vi "测试报告摘要4.vi"(8 "打印?":bool, 10 "试验时间":timestamp) -> ()   [LabVIEW 2010]
uses:
  <vilib>/Utility/NIReport.llb/NI_report.lvclass
  全局量/试验配置信息.vi
  <vilib>/Utility/NIReport.llb/Append Report Text (str wrap).vi
  全局量/自动测试结果.vi
  <vilib>/addons/_office/word.llb/Word Easy Table (str).vi
  <vilib>/addons/_office/NI_ReportGenerationToolkit.lvlib
panel:
  in  "序号":i32
  out "XY图":cluster{"Y":dbl[], "Y":dbl[]}[](graph)
  # "T：打印\nF：保存"
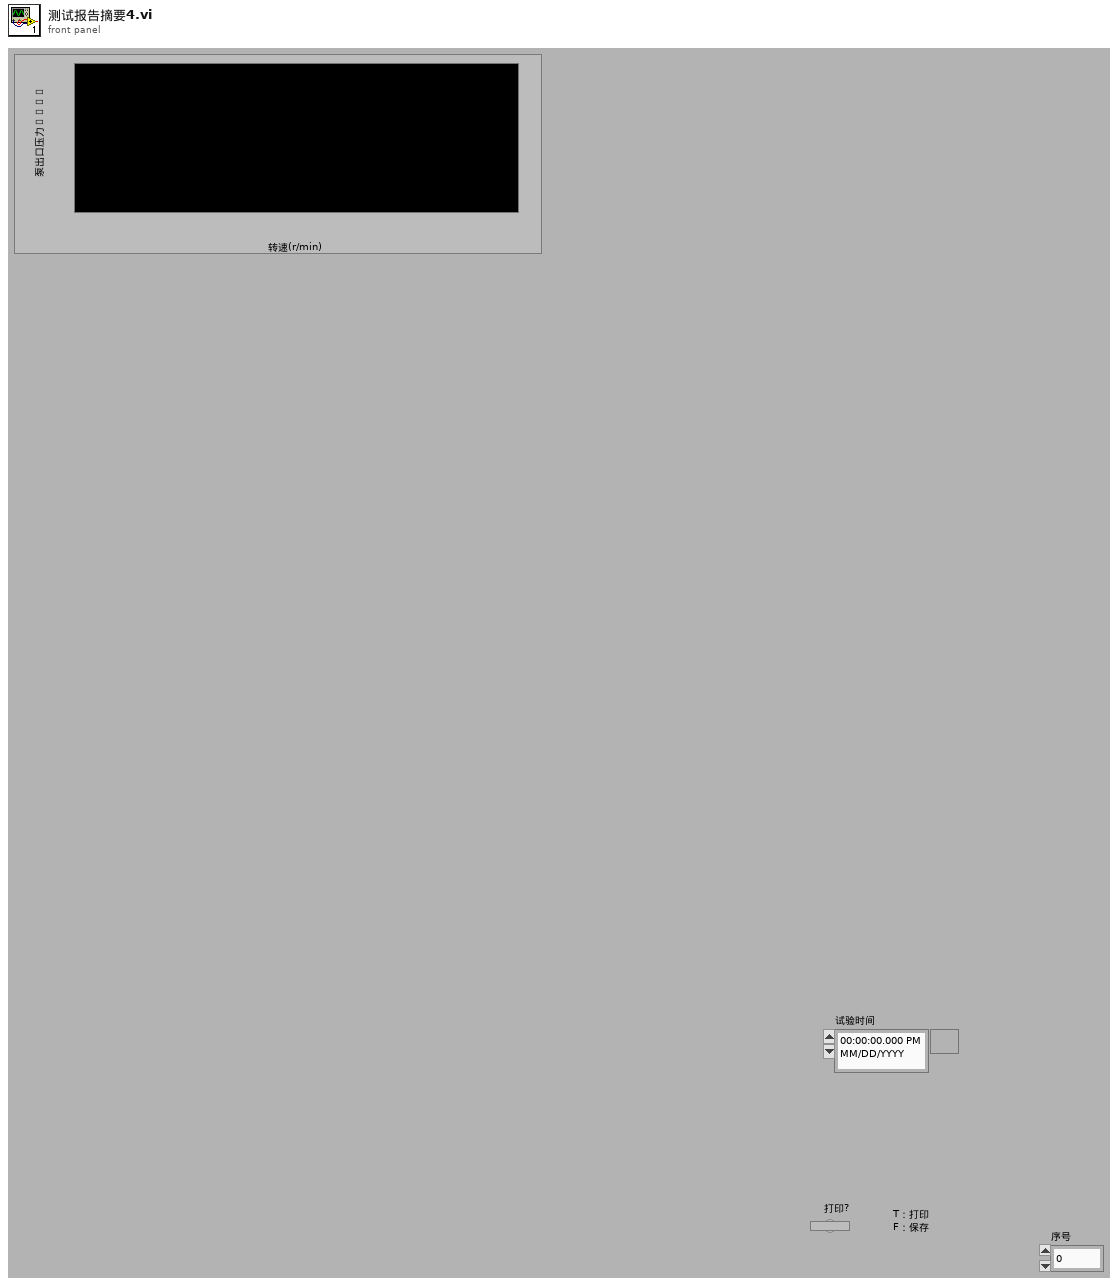
[diagram p1: front panel]
types:
  T1 = cluster{"position (Excel)":cluster{"row":i32, "column":i32}, "name (Excel)":string, "bookmark (Word)":string}
  T2 = enum16{"maximized", "minimized", "normal", "no change"}
  T3 = enum16{"Standard Report", "HTML", "Word", "Excel"}
  T4 = cluster{"报告编号":string, "控制板编号":string, "控制板类型":string, "测试人员":string, "测试地点":string, string, u64, "spreadsheet string":string, "spreadsheet string":string, "spreadsheet string":string, "spreadsheet string":string}
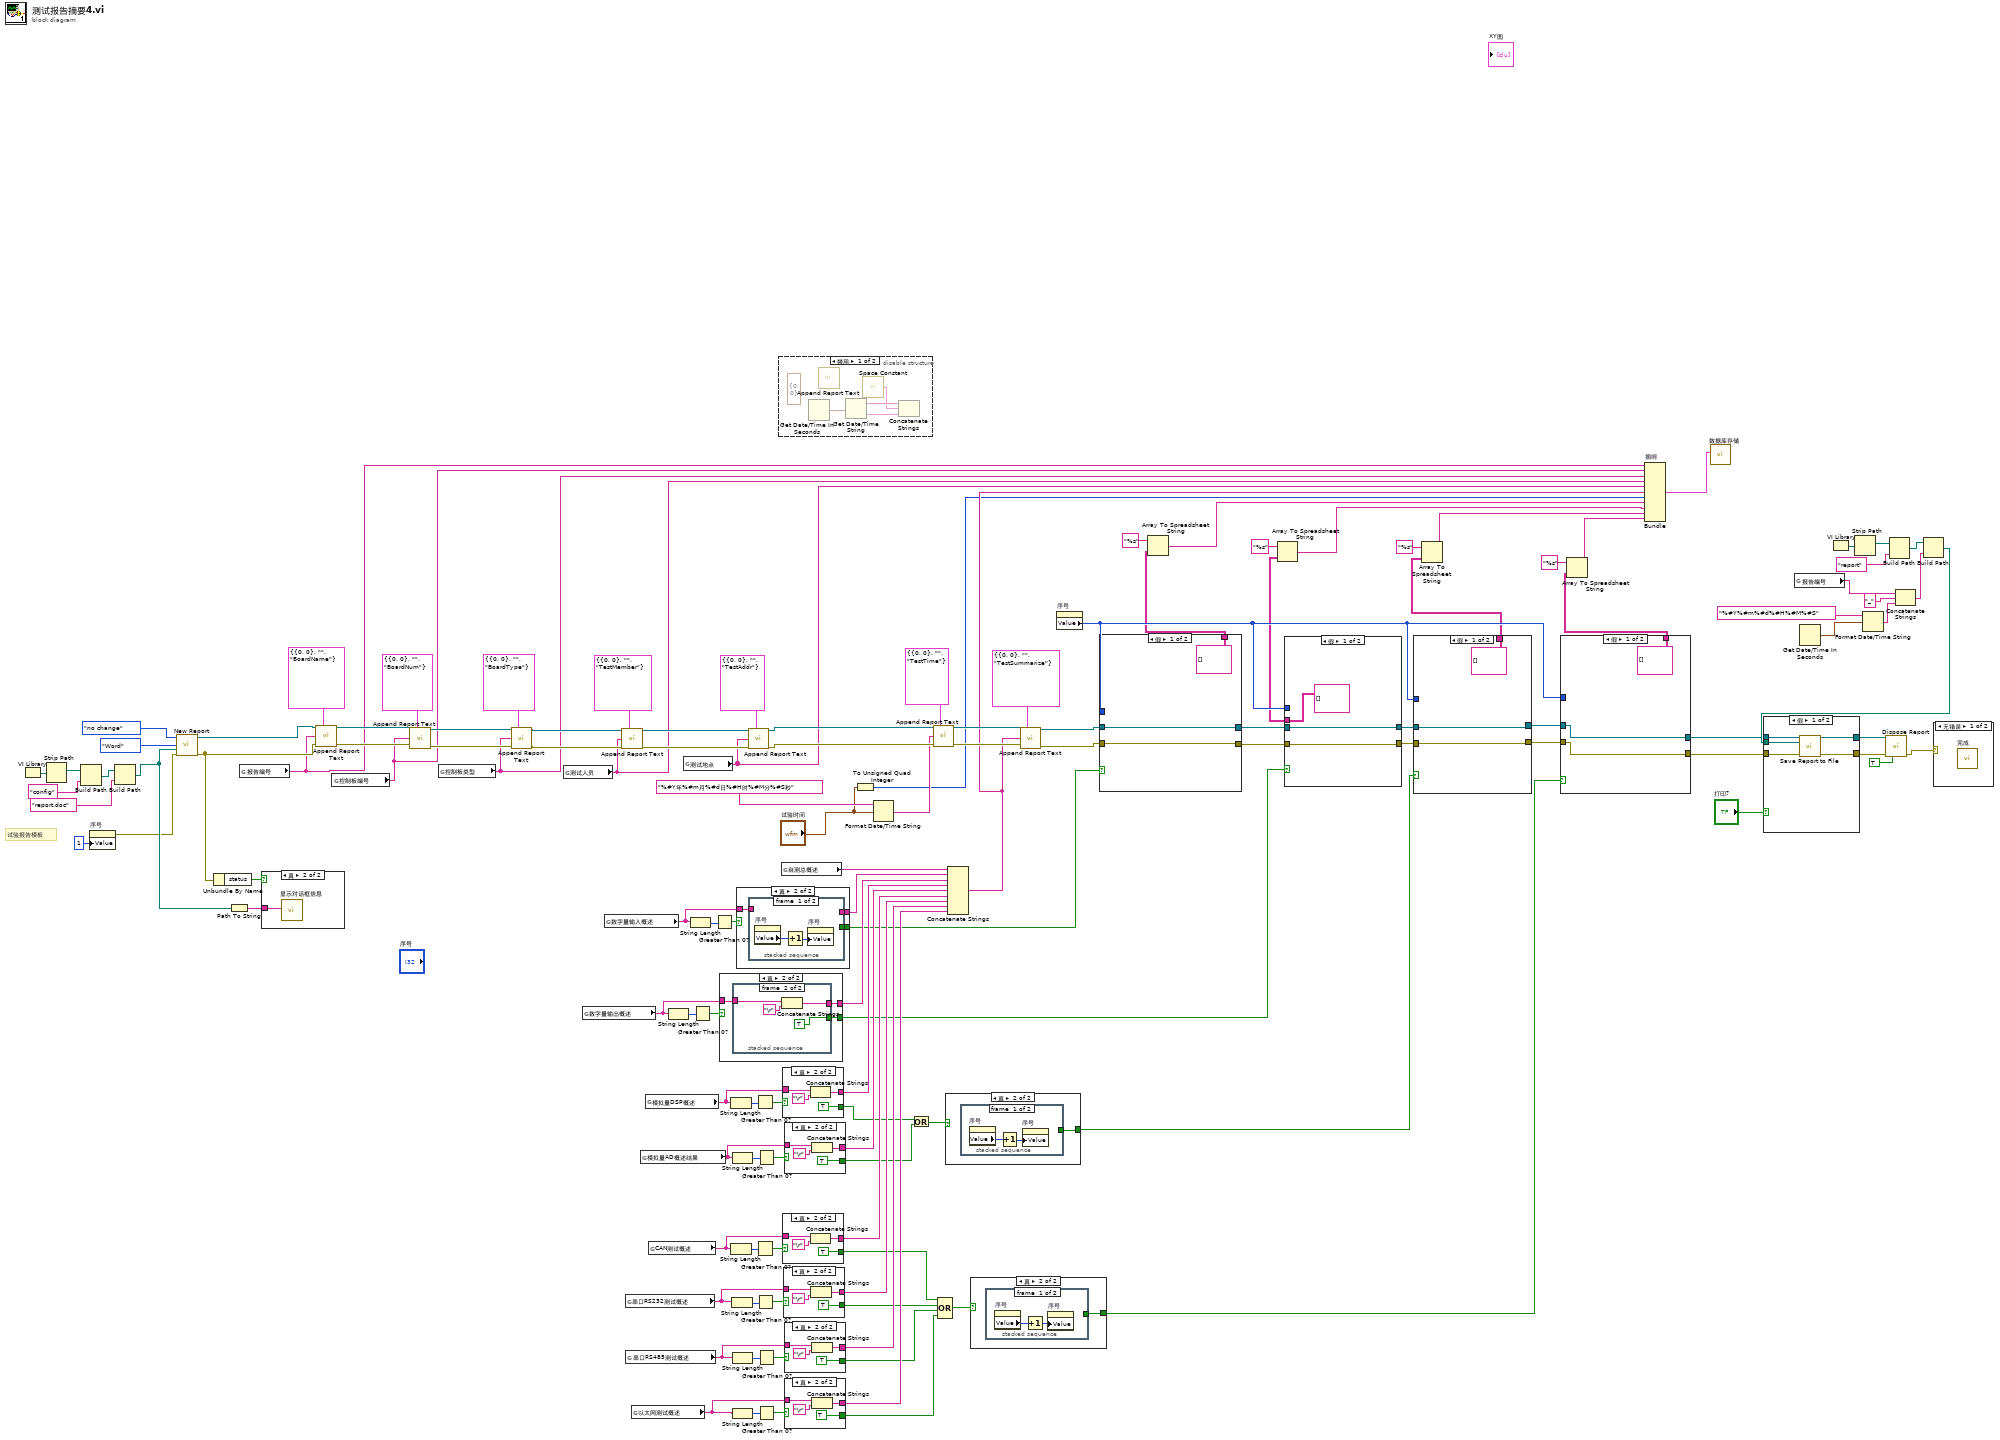
[diagram p0: block diagram]
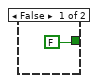
[diagram p2: hidden frame]
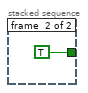
[diagram p3: hidden frame]
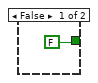
[diagram p4: hidden frame]
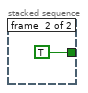
[diagram p5: hidden frame]
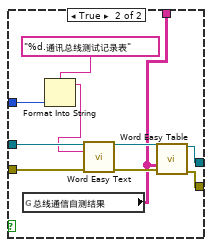
[diagram p6: hidden frame]
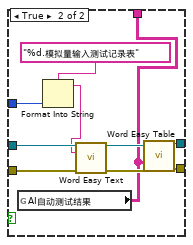
[diagram p7: hidden frame]
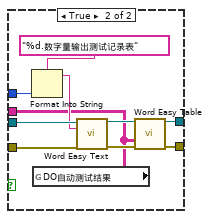
[diagram p8: hidden frame]
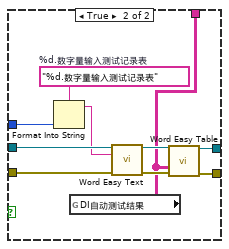
[diagram p9: hidden frame]
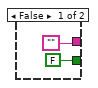
[diagram p10: hidden frame]
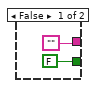
[diagram p11: hidden frame]
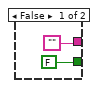
[diagram p12: hidden frame]
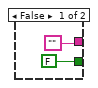
[diagram p13: hidden frame]
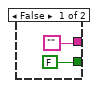
[diagram p14: hidden frame]
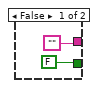
[diagram p15: hidden frame]
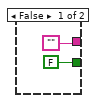
[diagram p16: hidden frame]
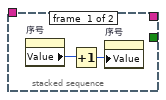
[diagram p17: hidden frame]
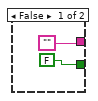
[diagram p18: hidden frame]
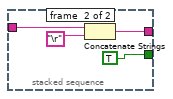
[diagram p19: hidden frame]
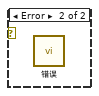
[diagram p20: hidden frame]
diagram:
  # "试验报告模板"
  n1 = VI Library() -> (path=w123:path)
  n2 = Strip Path(path=w123) -> (stripped path=w120:path)  [unwired: 1 out]
  n3 = Build Path(base path=w120, name or relative path="config") -> (appended path=w122:path)
  n4 = property on="序号" class="DigNum (严格)"("Value"=1 ("序号")) -> (error out=w40:errorcluster)  [unwired: 2 in, 1 out]
  n5 = Build Path(base path=w122, name or relative path="report.doc") -> (appended path=w126:path)
  n6 = call <vilib>:"New Report.vi"("window state (normal)"=T2."no change", "report type"=T3."Word", "template (empty)"=w126, "error in (no error)"=w40) -> ("report out"=w117:refnum<class "NI_report.lvclass">, "error out"=w116:errorcluster)  [unwired: 10 in]
  n7 = Unbundle By Name(w116) -> ("status"=w128:bool)
  n8 = Path To String(path=w126) -> (string=w127:string)
  n9 = global read "试验配置信息.vi" "报告编号"() -> (w20:string)
  n10 = case shown="真" w128 {
    tunnel: w127 -> [_ w129]
    frame False {
    }
    frame True {
      n11 = call "显示对话框信息"("Message"=w129) -> ()  [unwired: 9 in, 2 out]
    }
  }
  n12 = call-poly <vilib>:"Append Report Text.vi"("report in"=w117, "MS Office parameters"=T1 {"position (Excel)"={"row"=0, "column"=0}, "name (Excel)"="", "bookmark (Word)"="BoardName"}, "text"=w20, "error in (no error)"=w116) -> ("report out"=w102:refnum<class "NI_report.lvclass">, "error out"=w101:errorcluster)  [unwired: 8 in, 2 out]
  n13 = global read "试验配置信息.vi" "控制板编号"() -> (w19:string)
  n14 = call-poly <vilib>:"Append Report Text.vi"("report in"=w102, "MS Office parameters"=T1 {"position (Excel)"={"row"=0, "column"=0}, "name (Excel)"="", "bookmark (Word)"="BoardNum"}, "text"=w19, "error in (no error)"=w101) -> ("report out"=w112:refnum<class "NI_report.lvclass">, "error out"=w111:errorcluster)  [unwired: 8 in, 2 out]
  n15 = global read "试验配置信息.vi" "控制板类型"() -> (w18:string)
  n16 = call-poly <vilib>:"Append Report Text.vi"("report in"=w112, "MS Office parameters"=T1 {"position (Excel)"={"row"=0, "column"=0}, "name (Excel)"="", "bookmark (Word)"="BoardType"}, "text"=w18, "error in (no error)"=w111) -> ("report out"=w109:refnum<class "NI_report.lvclass">, "error out"=w108:errorcluster)  [unwired: 8 in, 2 out]
  n17 = global read "试验配置信息.vi" "测试人员"() -> (w17:string)
  n18 = global read "自动测试结果.vi" "数字量输出概述"() -> (w71:string)
  n19 = global read "自动测试结果.vi" "数字量输入概述"() -> (w72:string)
  n20 = call-poly <vilib>:"Append Report Text.vi"("report in"=w109, "MS Office parameters"=T1 {"position (Excel)"={"row"=0, "column"=0}, "name (Excel)"="", "bookmark (Word)"="TestMember"}, "text"=w17, "error in (no error)"=w108) -> ("report out"=w106:refnum<class "NI_report.lvclass">, "error out"=w105:errorcluster)  [unwired: 8 in, 2 out]
  n21 = global read "自动测试结果.vi" "串口RS232测试概述"() -> (w59:string)
  n22 = global read "自动测试结果.vi" "串口RS485测试概述"() -> (w54:string)
  n23 = global read "自动测试结果.vi" "以太网测试概述"() -> (w42:string)
  n24 = global read "自动测试结果.vi" "模拟量AD概述结果"() -> (w65:string)
  n25 = global read "自动测试结果.vi" "模拟量DSP概述"() -> (w66:string)
  n26 = global read "自动测试结果.vi" "CAN测试概述"() -> (w60:string)
  n27 = String Length(string=w71) -> (length=w69:i32)
  n28 = global read "试验配置信息.vi" "测试地点"() -> (w16:string)
  n29 = String Length(string=w72) -> (length=w74:i32)
  n30 = Greater Than 0?(x=w69) -> (x > 0?=w70:bool)
  n31 = Greater Than 0?(x=w74) -> (x > 0?=w73:bool)
  n32 = case shown="真" w70 {
    tunnel: w71 -> [_ w134]
    tunnel: ["" w133] -> w50
    tunnel: [FALSE w132] -> w38
    frame False {
    }
    frame True {
      n33 = stacked-sequence {
        tunnel: w134 -> [_ w140]
        tunnel: [_ w138] -> w133
        tunnel: [_ TRUE] -> w132
        frame #0 {
          n34 = property on="序号" class="DigNum (严格)"() -> ("Value"=w136:i32)  [unwired: 2 in, 2 out]
          n35 = Increment(x=w136) -> (x+1=w135:i32)
          n36 = property on="序号" class="DigNum (严格)"("Value"=w135) -> ()  [unwired: 2 in, 2 out]
        }
        frame #1 {
          n37 = Concatenate Strings(w140, "\r") -> (w138:string)
        }
      }
    }
  }
  n38 = String Length(string=w66) -> (length=w68:i32)
  n39 = String Length(string=w60) -> (length=w62:i32)
  n40 = String Length(string=w59) -> (length=w57:i32)
  n41 = String Length(string=w65) -> (length=w63:i32)
  n42 = String Length(string=w54) -> (length=w56:i32)
  n43 = String Length(string=w42) -> (length=w53:i32)
  n44 = case shown="真" w73 {
    tunnel: w72 -> [_ w145]
    tunnel: ["" w144] -> w51
    tunnel: [FALSE w143] -> w39
    frame False {
    }
    frame True {
      n45 = stacked-sequence {
        tunnel: w145 -> [_ w151]
        tunnel: [_ w149] -> w144
        tunnel: [_ TRUE] -> w143
        frame #0 {
          n46 = property on="序号" class="DigNum (严格)"() -> ("Value"=w146:i32)  [unwired: 2 in, 2 out]
          n47 = Increment(x=w146) -> (x+1=w147:i32)
          n48 = property on="序号" class="DigNum (严格)"("Value"=w147) -> ()  [unwired: 2 in, 2 out]
        }
        frame #1 {
          n49 = Concatenate Strings(w151, "\r") -> (w149:string)
        }
      }
    }
  }
  n50 = call-poly <vilib>:"Append Report Text.vi"("report in"=w106, "MS Office parameters"=T1 {"position (Excel)"={"row"=0, "column"=0}, "name (Excel)"="", "bookmark (Word)"="TestAddr"}, "text"=w16, "error in (no error)"=w105) -> ("report out"=w104:refnum<class "NI_report.lvclass">, "error out"=w103:errorcluster)  [unwired: 8 in, 2 out]
  n51 = Greater Than 0?(x=w68) -> (x > 0?=w67:bool)
  n52 = Greater Than 0?(x=w62) -> (x > 0?=w61:bool)
  n53 = Greater Than 0?(x=w57) -> (x > 0?=w58:bool)
  n54 = Greater Than 0?(x=w63) -> (x > 0?=w64:bool)
  n55 = Greater Than 0?(x=w56) -> (x > 0?=w55:bool)
  n56 = Greater Than 0?(x=w53) -> (x > 0?=w43:bool)
  n57 = disable-structure shown="禁用" {
    frame Disabled {
      (unwired) cluster{"row":i32, "column":i32} {"row"=0, "column"=0} ("position (excel)")
      n58 = Get Date/Time In Seconds() -> (seconds since 1Jan1904=w155:timestamp)
      n59 = call-poly <vilib>:"Append Report Text.vi"() -> ()  [unwired: 12 in, 4 out]
      n60 = Get Date/Time String(seconds (now)=w155) -> (date string=w154:string, time string=w153:string)  [unwired: 2 in]
      n61 = call <vilib>:"Space Constant.vi"() -> ("String"=w152:string)
      n62 = Concatenate Strings(w154, w152, w153) -> ()  [unwired: 1 out]
    }
    frame Enabled {
    }
  }
  n63 = global read "自动测试结果.vi" "自测总概述"() -> (w52:string)
  n64 = case shown="真" w67 {
    tunnel: w66 -> [_ w161]
    tunnel: ["" w159] -> w49
    tunnel: [FALSE TRUE] -> w37
    frame False {
    }
    frame True {
      n65 = Concatenate Strings(w161, "\r") -> (w159:string)
    }
  }
  n66 = case shown="真" w61 {
    tunnel: w60 -> [_ w167]
    tunnel: ["" w165] -> w47
    tunnel: [FALSE TRUE] -> w34
    frame False {
    }
    frame True {
      n67 = Concatenate Strings(w167, "\r") -> (w165:string)
    }
  }
  n68 = case shown="真" w58 {
    tunnel: w59 -> [_ w173]
    tunnel: ["" w171] -> w46
    tunnel: [FALSE TRUE] -> w33
    frame False {
    }
    frame True {
      n69 = Concatenate Strings(w173, "\r") -> (w171:string)
    }
  }
  n70 = case shown="真" w64 {
    tunnel: w65 -> [_ w179]
    tunnel: ["" w177] -> w48
    tunnel: [FALSE TRUE] -> w36
    frame False {
    }
    frame True {
      n71 = Concatenate Strings(w179, "\r") -> (w177:string)
    }
  }
  n72 = case shown="真" w55 {
    tunnel: w54 -> [_ w185]
    tunnel: ["" w183] -> w45
    tunnel: [FALSE TRUE] -> w32
    frame False {
    }
    frame True {
      n73 = Concatenate Strings(w185, "\r") -> (w183:string)
    }
  }
  n74 = case shown="真" w43 {
    tunnel: w42 -> [_ w191]
    tunnel: ["" w189] -> w44
    tunnel: [FALSE TRUE] -> w31
    frame False {
    }
    frame True {
      n75 = Concatenate Strings(w191, "\r") -> (w189:string)
    }
  }
  n76 = To Unsigned Quad Integer(1:"试验时间") -> (0:w14:u64)
  n77 = Format Date/Time String(time format string (%c)="%#Y年%#m月%#d日%#H时%#M分%#S秒" ("时间格式字符串(%c)"), seconds (now)="试验时间") -> (date/time string=w22:string)  [unwired: 1 in]
  n78 = Or(x=w37, y=w36) -> (x .or. y?=w35:bool)
  n79 = call-poly <vilib>:"Append Report Text.vi"("report in"=w104, "MS Office parameters"=T1 {"position (Excel)"={"row"=0, "column"=0}, "name (Excel)"="", "bookmark (Word)"="TestTime"}, "text"=w22, "error in (no error)"=w103) -> ("report out"=w78:refnum<class "NI_report.lvclass">, "error out"=w77:errorcluster)  [unwired: 8 in, 2 out]
  n80 = Compound Arithmetic op=OR(w34, w33, w32, w31) -> (w30:bool)
  n81 = case shown="真" w35 {
    tunnel: [FALSE w193] -> w29
    frame False {
    }
    frame True {
      n82 = stacked-sequence {
        tunnel: [_ TRUE] -> w193
        frame #0 {
          n83 = property on="序号" class="DigNum (严格)"() -> ("Value"=w195:i32)  [unwired: 2 in, 2 out]
          n84 = Increment(x=w195) -> (x+1=w194:i32)
          n85 = property on="序号" class="DigNum (严格)"("Value"=w194) -> ()  [unwired: 2 in, 2 out]
        }
        frame #1 {
        }
      }
    }
  }
  n86 = Concatenate Strings(w52, w51, w50, w49, w48, w47, w46, w45, w44) -> (w15:string)
  n87 = case shown="真" w30 {
    tunnel: [FALSE w198] -> w27
    frame False {
    }
    frame True {
      n88 = stacked-sequence {
        tunnel: [_ TRUE] -> w198
        frame #0 {
          n89 = property on="序号" class="DigNum (严格)"() -> ("Value"=w200:i32)  [unwired: 2 in, 2 out]
          n90 = Increment(x=w200) -> (x+1=w199:i32)
          n91 = property on="序号" class="DigNum (严格)"("Value"=w199) -> ()  [unwired: 2 in, 2 out]
        }
        frame #1 {
        }
      }
    }
  }
  n92 = call-poly <vilib>:"Append Report Text.vi"("report in"=w78, "MS Office parameters"=T1 {"position (Excel)"={"row"=0, "column"=0}, "name (Excel)"="", "bookmark (Word)"="TestSummarize"}, "text"=w15, "error in (no error)"=w77) -> ("report out"=w76:refnum<class "NI_report.lvclass">, "error out"=w75:errorcluster)  [unwired: 8 in, 2 out]
  n93 = property on="序号" class="DigNum (严格)"() -> ("Value"=w28:i32)  [unwired: 2 in, 2 out]
  n94 = case shown="假" w39 {
    tunnel: [w204 w213] -> w86
    tunnel: [w203 w212] -> w84
    tunnel: w76 -> [w204 w210]
    tunnel: w75 -> [w203 w209]
    tunnel: w28 -> [_ w206]
    tunnel: [string[][] [] ("DI自动测试结果") w205] -> w12
    frame False {
    }
    frame True {
      w208 = "%d.数字量输入测试记录表"  # %d.数字量输入测试记录表
      n95 = Format Into String(format string=w208, w206) -> (resulting string=w207:string)  [unwired: 2 in, 1 out]
      n96 = global read "自动测试结果.vi" "DI自动测试结果"() -> (w205:string[][])
      n97 = call <vilib>:"Word Easy Text.vi"("report in"=w210, "text"=w207, "error in (no error)"=w209) -> ("report out"=w214:refnum<class "NI_report.lvclass">, "error out"=w211:errorcluster)  [unwired: 10 in, 1 out]
      n98 = call-poly <vilib>:"Word Easy Table.vi"("report in"=w214, "data"=w205, "error in (no error)"=w211) -> ("report out"=w213:refnum<class "NI_report.lvclass">, "error out"=w212:errorcluster)  [unwired: 10 in, 1 out]
    }
  }
  n99 = Array To Spreadsheet String(array=w12, 3:"%s" ("格式字符串")) -> (spreadsheet string=w11:string)  [unwired: 1 in]
  n100 = case shown="假" w38 {
    tunnel: w86 -> [w217 w227]
    tunnel: [w217 w225] -> w85
    tunnel: w84 -> [w216 w224]
    tunnel: [w216 w222] -> w83
    tunnel: w28 -> [_ w220]
    tunnel: [string[][] [] ("DO自动测试结果") w218] -> w9
    frame False {
    }
    frame True {
      n101 = Format Into String(format string="%d.数字量输出测试记录表", w220) -> (resulting string=w219:string)  [unwired: 2 in, 1 out]
      n102 = global read "自动测试结果.vi" "DO自动测试结果"() -> (w218:string[][])
      n103 = call <vilib>:"Word Easy Text.vi"("report in"=w227, "text"=w219, "error in (no error)"=w224) -> ("report out"=w226:refnum<class "NI_report.lvclass">, "error out"=w223:errorcluster)  [unwired: 10 in, 1 out]
      n104 = call-poly <vilib>:"Word Easy Table.vi"("report in"=w226, "data"=w218, "error in (no error)"=w223) -> ("report out"=w225:refnum<class "NI_report.lvclass">, "error out"=w222:errorcluster)  [unwired: 10 in, 1 out]
    }
  }
  n105 = Array To Spreadsheet String(array=w9, 3:"%s" ("格式字符串")) -> (spreadsheet string=w8:string)  [unwired: 1 in]
  n106 = case shown="假" w29 {
    tunnel: w85 -> [w230 w240]
    tunnel: w83 -> [w229 w238]
    tunnel: [w230 w236] -> w82
    tunnel: [w229 w235] -> w81
    tunnel: w28 -> [_ w233]
    tunnel: [string[][] [] ("AI自动测试结果") w231] -> w6
    frame False {
    }
    frame True {
      n107 = global read "自动测试结果.vi" "AI自动测试结果"() -> (w231:string[][])
      n108 = Format Into String(format string="%d.模拟量输入测试记录表", w233) -> (resulting string=w232:string)  [unwired: 2 in, 1 out]
      n109 = call <vilib>:"Word Easy Text.vi"("report in"=w240, "text"=w232, "error in (no error)"=w238) -> ("report out"=w239:refnum<class "NI_report.lvclass">, "error out"=w237:errorcluster)  [unwired: 10 in, 1 out]
      n110 = call-poly <vilib>:"Word Easy Table.vi"("report in"=w239, "data"=w231, "error in (no error)"=w237) -> ("report out"=w236:refnum<class "NI_report.lvclass">, "error out"=w235:errorcluster)  [unwired: 10 in, 1 out]
    }
  }
  n111 = Array To Spreadsheet String(array=w6, 3:"%s" ("格式字符串")) -> (spreadsheet string=w5:string)  [unwired: 1 in]
  n112 = case shown="假" w27 {
    tunnel: [w243 w253] -> w88
    tunnel: [w242 w252] -> w87
    tunnel: w82 -> [w243 w251]
    tunnel: w81 -> [w242 w250]
    tunnel: w28 -> [_ w246]
    tunnel: [string[][] [] ("总线通信自测结果") w244] -> w3
    frame False {
    }
    frame True {
      n113 = global read "自动测试结果.vi" "总线通信自测结果"() -> (w244:string[][])
      n114 = Format Into String(format string="%d.通讯总线测试记录表", w246) -> (resulting string=w245:string)  [unwired: 2 in, 1 out]
      n115 = call <vilib>:"Word Easy Text.vi"("report in"=w251, "text"=w245, "error in (no error)"=w250) -> ("report out"=w249:refnum<class "NI_report.lvclass">, "error out"=w248:errorcluster)  [unwired: 10 in, 1 out]
      n116 = call-poly <vilib>:"Word Easy Table.vi"("report in"=w249, "data"=w244, "error in (no error)"=w248) -> ("report out"=w253:refnum<class "NI_report.lvclass">, "error out"=w252:errorcluster)  [unwired: 10 in, 1 out]
    }
  }
  n117 = Array To Spreadsheet String(array=w3, 3:"%s" ("格式字符串")) -> (spreadsheet string=w2:string)  [unwired: 1 in]
  n118 = Bundle "捆绑"("报告编号"=w20, "控制板编号"=w19, "控制板类型"=w18, "测试人员"=w17, "测试地点"=w16, w15, w14, "spreadsheet string"=w11, "spreadsheet string"=w8, "spreadsheet string"=w5, "spreadsheet string"=w2) -> (w1:T4)  [unwired: 1 in]
  n119 = call "数据库存储.vi"("输出簇 2"=w1) -> ()  [unwired: 10 in]
  n120 = global read "试验配置信息.vi" "报告编号"() -> (w25:string)
  n121 = Get Date/Time In Seconds() -> (seconds since 1Jan1904=w95:timestamp)
  n122 = VI Library() -> (path=w96:path)
  n123 = Strip Path(path=w96) -> (stripped path=w99:path)  [unwired: 1 out]
  n124 = Format Date/Time String(time format string (%c)="%#Y%#m%#d%#H%#M%#S" ("时间格式字符串(%c)"), seconds (now)=w95) -> (date/time string=w26:string)  [unwired: 1 in]
  n125 = Build Path(base path=w99, name or relative path="report") -> (appended path=w97:path)
  n126 = Concatenate Strings(w25, "_", w26) -> (w23:string)
  n127 = Build Path(base path=w97, name or relative path=w23) -> (appended path=w90:path)
  n128 = case shown="假" "打印?" {
    tunnel: w88 -> [w258 w262]
    tunnel: w87 -> [w257 w261]
    tunnel: [w256 w260] -> w93
    tunnel: [w255 w259] -> w92
    tunnel: w90 -> [w254 _]
    frame False {
      n129 = call-dynamic "Save Report to File.vi"("report in"=w258, "report file path"=w254, "error in (no error)"=w257) -> ("report out"=w256:refnum<class "NI_report.lvclass">, "error out"=w255:errorcluster)  [unwired: 11 in]
    }
    frame True {
      n130 = call-dynamic "Print Report.vi"("report in"=w262, "error in (no error)"=w261) -> ("report out"=w260:refnum<class "NI_report.lvclass">, "error out"=w259:errorcluster)  [unwired: 12 in]
    }
  }
  n131 = call-dynamic "Dispose Report.vi"("report in"=w93, "error in (no error)"=w92, "close report? (T)"=TRUE) -> ("error out"=w89:errorcluster)  [unwired: 12 in]
  n132 = case shown="无错误" w89 {
    frame No Error {
      n133 = call "完成"() -> ()  [unwired: 10 in, 2 out]
    }
    frame Error {
      n134 = call "错误"() -> ()  [unwired: 10 in, 2 out]
    }
  }
